vi "Enable Cycling.vi"(8 "error in (no error)":errorcluster, 11 "Data Cluster in":T1 {"VestaTemperature"."Water Heater Temp (°F)" min=32 max=203}) -> (0 "error out":errorcluster, 3 "Data Cluster out":T1 {"VestaTemperature"."Water Heater Temp (°F)" min=32 max=203}, 4 "Send_Vesta_Message":u8, 6 "Send_Timer_Message":u8)   [LabVIEW 2023]
uses:
  Drivers/Resideo Gas Valve/Type Definitions/Vesta Info.ctl
  controls/Burner Duty Cycle.ctl
  Drivers/Resideo Gas Valve/Type Definitions/Temperature Control.ctl
  controls/UI Data.ctl
  controls/Timer Application Cluster.ctl
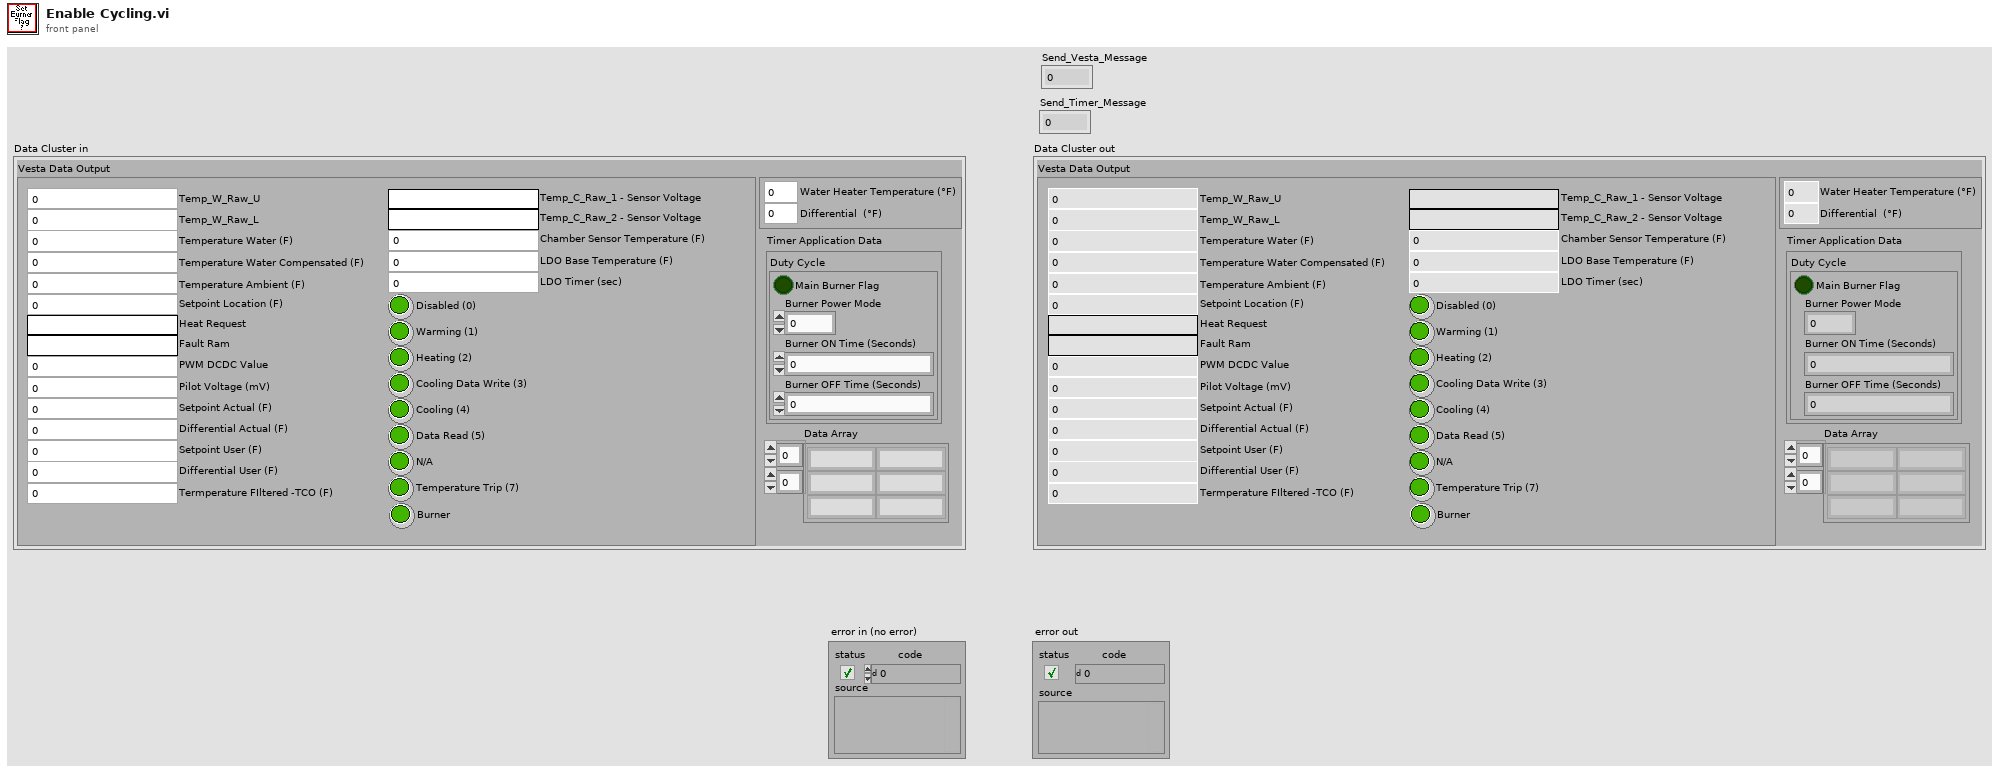
[diagram p1: front panel]
types:
  T1 = typedef "UI Data.ctl" = cluster{"Vesta Data Output":T2, "VestaTemperature":T3, "Timer Application Data":T4, "Data Array":string[][]}
  T2 = typedef "Vesta Info.ctl" = cluster{"Temp_W_Raw_U":u16, "Temp_W_Raw_L":u16, "Temperature Water (F)":dbl, "Temperature Water Compensated (F)":dbl, "Temperature Ambient (F)":dbl, "Setpoint Location (F)":dbl, "Heat Request":string, "Fault Ram":string, "PWM DCDC Value":u16, "Pilot Voltage (mV)":dbl, "Setpoint Actual (F)":dbl, "Differential Actual (F)":dbl, "Setpoint User (F)":dbl, "Differential User (F)":dbl, "Termperature FIltered -TCO (F)":dbl, "Temp_C_Raw_1 - Sensor Voltage":string, "Temp_C_Raw_2 - Sensor Voltage":string, "Chamber Sensor Temperature (F)":dbl, "LDO Base Temperature (F)":dbl, "LDO Timer (sec)":i16, "Disabled (0)":bool, "Warming (1)":bool, "Heating (2)":bool, "Cooling Data Write (3)":bool, "Cooling (4)":bool, "Data Read (5)":bool, "N/A":bool, "Temperature Trip (7)":bool, "Burner":bool}
  T3 = typedef "Temperature Control.ctl" = cluster{"Water Heater Temp (°F)":u16, "Differential  (°F)":dbl}
  T4 = typedef "Timer Application Cluster.ctl" = cluster{"Duty Cycle":T5}
  T5 = typedef "Burner Duty Cycle.ctl" = cluster{"Burner ON Time (Seconds)":dbl, "Burner OFF Time (Seconds)":dbl, "Main Burner Flag":bool, "Burner Power Mode":u8}
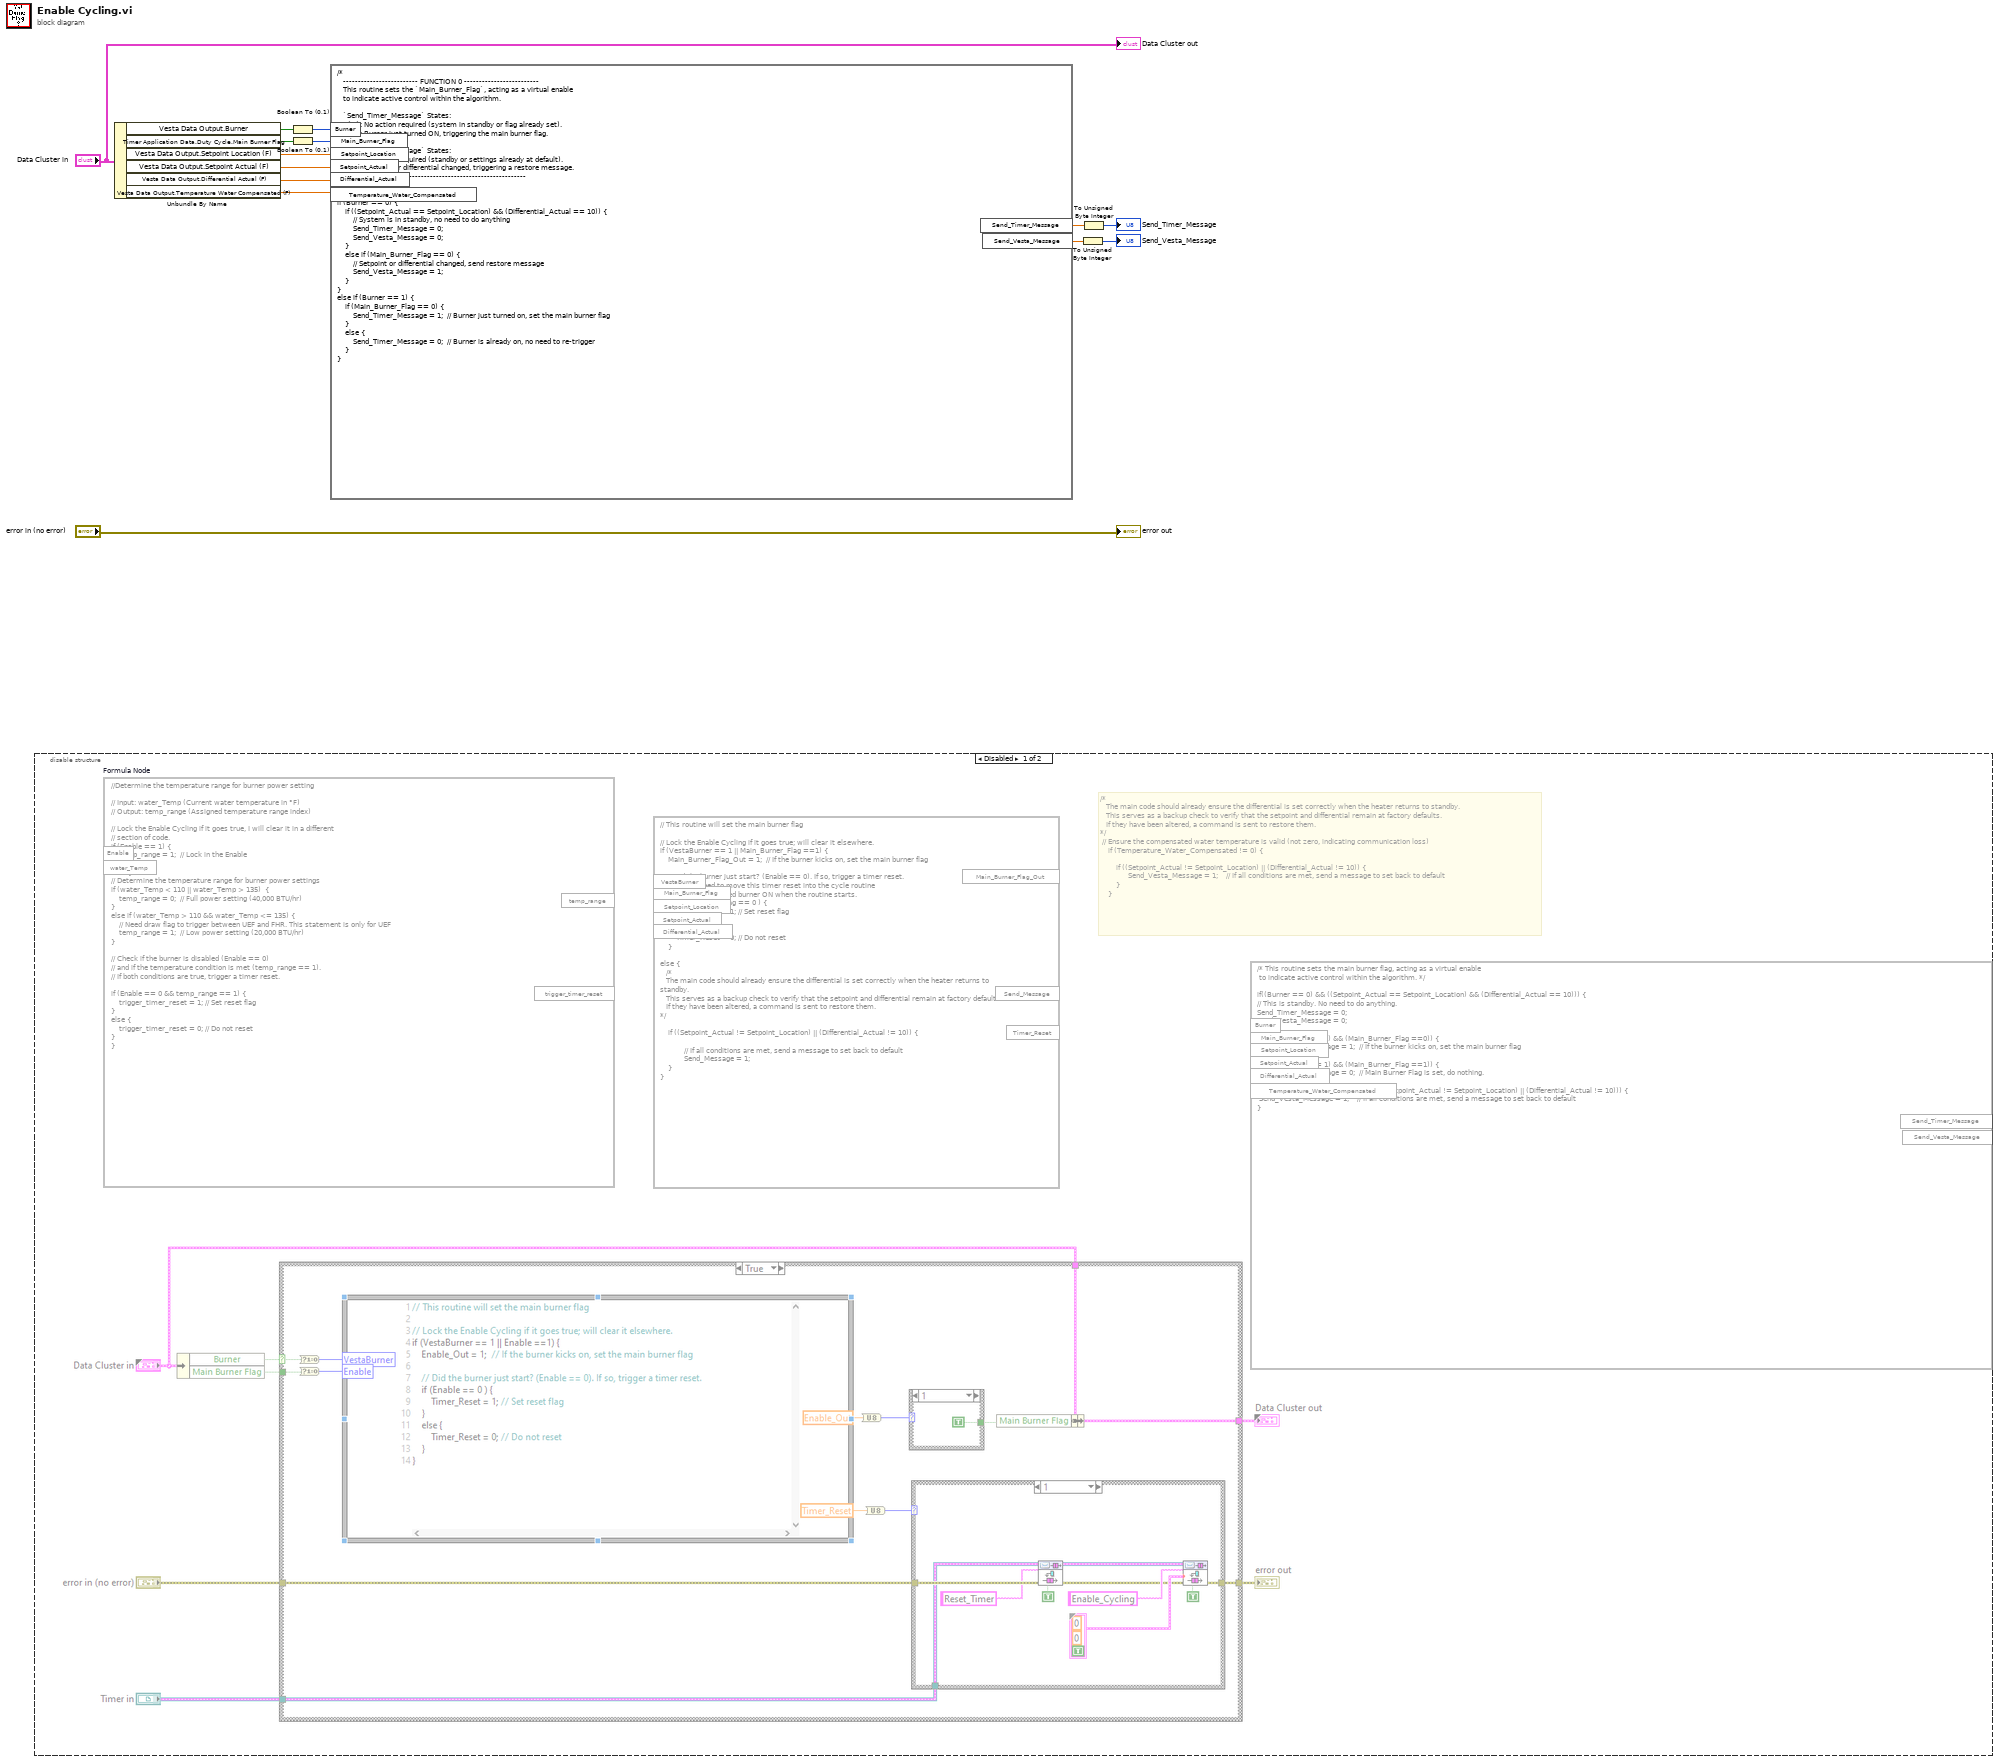
[diagram p0: block diagram]
diagram:
  n1 = disable-structure shown="Disabled" {
    frame Disabled {
      # "/* \n   The main code should already ensure the differential is set correctly when the heater returns to standby.  \n   This serves as a backup check to verify that the setpoint and differential remain at factory defaults.  \n   If they have been altered, a command is sent to restore them.  \n*/\n // Ensure the compensated water temperature is valid (not zero, indicating communication loss)\n    if (Temperature_Water_Compensated != 0) {  \n\n        if ((Setpoint_Actual != Setpoint_Location) || (Differential_Actual != 10)) {                 \n              Send_Vesta_Message = 1;    // If all conditions are met, send a message to set back to default \n        }\n    }"
      n2 = formula code="//Determine the temperature range for burner power setting\n\n// Input: water_Temp (Current water temperature in °F)\n// Output: temp_range (Assigned temperature range index)\n\n// Lock the Enable Cycling if it goes true, I will clear it in a different\n// section of code.\nif (Enable == 1) {\n    temp_range = 1;  // Lock in the Enable\n}\nelse {\n// Determine the temperature range for burner power settings\nif (water_Temp < 110 || water_Temp > 135)  {\n    temp_range = 0;  // Full power setting (40,000 BTU/hr)\n} \nelse if (water_Temp > 110 && water_Temp <= 135) {\n    // Need draw flag to trigger between UEF and FHR. This statement is only for UEF\n    temp_range = 1;  // Low power setting (20,000 BTU/hr)\n} \n\n// Check if the burner is disabled (Enable == 0) \n// and if the temperature condition is met (temp_range == 1).\n// If both conditions are true, trigger a timer reset.\n\nif (Enable == 0 && temp_range == 1) { \n    trigger_timer_reset = 1; // Set reset flag\n}\nelse { \n    trigger_timer_reset = 0; // Do not reset\n}\n}"() -> ()  [unwired: 2 in, 2 out]
      n3 = formula code="// This routine will set the main burner flag\n\n// Lock the Enable Cycling if it goes true; will clear it elsewhere.\nif (VestaBurner == 1 || Main_Burner_Flag ==1) {\n    Main_Burner_Flag_Out = 1;  // If the burner kicks on, set the main burner flag\n\n    // Did the burner just start? (Enable == 0). If so, trigger a timer reset.\n    // I really need to move this timer reset into the cycle routine\n   // this is for a defined burner ON when the routine starts. \n   if (Main_Burner_Flag == 0 ) { \n        Timer_Reset = 1; // Set reset flag\n    }\n    else { \n        Timer_Reset = 0; // Do not reset\n    }   \n\nelse {\n   /* \n   The main code should already ensure the differential is set correctly when the heater returns to standby.  \n   This serves as a backup check to verify that the setpoint and differential remain at factory defaults.  \n   If they have been altered, a command is sent to restore them.  \n*/\n\n    if ((Setpoint_Actual != Setpoint_Location) || (Differential_Actual != 10)) {             \n            \n            // If all conditions are met, send a message to set back to default\n            Send_Message = 1;  \n    }\n}"() -> ()  [unwired: 5 in, 3 out]
      n4 = formula code="/* This routine sets the main burner flag, acting as a virtual enable  \n to indicate active control within the algorithm. */ \n\nif((Burner == 0) && ((Setpoint_Actual == Setpoint_Location) && (Differential_Actual == 10))) {\n// This is standby. No need to do anything.\nSend_Timer_Message = 0;\nSend_Vesta_Message = 0;\n}\nelse if ((Burner == 1) && (Main_Burner_Flag ==0)) {\n    Send_Timer_Message = 1;  // If the burner kicks on, set the main burner flag\n}\nelse if ((Burner == 1) && (Main_Burner_Flag ==1)) {\n    Send_Timer_Message = 0;  // Main Burner Flag is set, do nothing.\n}\nelse if ((Main_Burner_Flag ==0) && ((Setpoint_Actual != Setpoint_Location) || (Differential_Actual != 10))) {\n Send_Vesta_Message = 1;    // If all conditions are met, send a message to set back to default \n}"() -> ()  [unwired: 6 in, 2 out]
    }
    frame Enabled {
    }
  }
  n5 = Unbundle By Name("Data Cluster in") -> ("Vesta Data Output.Burner"=w13:bool, "Timer Application Data.Duty Cycle.Main Burner Flag"=w14:bool, "Vesta Data Output.Setpoint Location (F)"=w9:dbl, "Vesta Data Output.Setpoint Actual (F)"=w8:dbl, "Vesta Data Output.Differential Actual (F)"=w7:dbl, "Vesta Data Output.Temperature Water Compensated (F)"=w5:dbl)
  n6 = Boolean To (0,1)(Boolean=w13) -> (0, 1=w10:i16)
  n7 = Boolean To (0,1)(Boolean=w14) -> (0, 1=w11:i16)
  n8 = formula code="/*  \n   ------------------------- FUNCTION 0 -------------------------  \n   This routine sets the `Main_Burner_Flag`, acting as a virtual enable  \n   to indicate active control within the algorithm.  \n   \n   `Send_Timer_Message` States:  \n   - `0`: No action required (system in standby or flag already set).  \n   - `1`: Burner just turned ON, triggering the main burner flag.  \n\n   `Send_Vesta_Message` States:  \n   - `0`: No action required (standby or settings already at default).  \n   - `1`: Setpoint or differential changed, triggering a restore message.  \n   -------------------------------------------------------------  \n*/\n\nif (Burner == 0) {\n    if ((Setpoint_Actual == Setpoint_Location) && (Differential_Actual == 10)) {\n        // System is in standby, no need to do anything\n        Send_Timer_Message = 0;\n        Send_Vesta_Message = 0;\n    } \n    else if (Main_Burner_Flag == 0) {\n        // Setpoint or differential changed, send restore message\n        Send_Vesta_Message = 1;\n    }\n} \nelse if (Burner == 1) {\n    if (Main_Burner_Flag == 0) {\n        Send_Timer_Message = 1;  // Burner just turned on, set the main burner flag\n    } \n    else {\n        Send_Timer_Message = 0;  // Burner is already on, no need to re-trigger\n    }\n}"("Main_Burner_Flag"=w11, "Burner"=w10, "Setpoint_Location"=w9, "Setpoint_Actual"=w8, "Differential_Actual"=w7, "Temperature_Water_Compensated"=w5) -> ("Send_Timer_Message"=w12:dbl, "Send_Vesta_Message"=w6:dbl)
  n9 = To Unsigned Byte Integer(number=w6) -> (unsigned 8bit integer=→"Send_Vesta_Message":u8)
  n10 = To Unsigned Byte Integer(number=w12) -> (unsigned 8bit integer=→"Send_Timer_Message":u8)
  "Data Cluster out" <- "Data Cluster in"
  "error out" <- "error in (no error)"
